vi "FipsAdjacent.vi"() -> (11 "Fips":i32[](array[numeric]))   [LabVIEW 2017] (continued)
\t33013\n\"Merrimack County, NH\"\t33013\t\"Rockingham County, NH\"\t33015\n\"Merrimack County, NH\"\t33013\t\"Strafford County, NH\"\t33017\n\"Merrimack County, NH\"\t33013\t\"Sullivan County, NH\"\t33019\n\"Rockingham County, NH\"\t33015\t\"York County, ME\"\t23031\n\"Rockingham County, NH\"\t33015\t\"Essex County, MA\"\t25009\n\"Rockingham County, NH\"\t33015\t\"Hillsborough County, NH\"\t33011\n\"Rockingham County, NH\"\t33015\t\"Merrimack County, NH\"\t33013\n\"Rockingham County, NH\"\t33015\t\"Rockingham County, NH\"\t33015\n\"Rockingham County, NH\"\t33015\t\"Strafford County, NH\"\t33017\n\"Strafford County, NH\"\t33017\t\"York County, ME\"\t23031\n\"Strafford County, NH\"\t33017\t\"Belknap County, NH\"\t33001\n\"Strafford County, NH\"\t33017\t\"Carroll County, NH\"\t33003\n\"Strafford County, NH\"\t33017\t\"Merrimack County, NH\"\t33013\n\"Strafford County, NH\"\t33017\t\"Rockingham County, NH\"\t33015\n\"Strafford County, NH\"\t33017\t\"Strafford County, NH\"\t33017\n\"Sullivan County, NH\"\t33019\t\"Cheshire County, NH\"\t33005\n\"Sullivan County, NH\"\t33019\t\"Grafton County, NH\"\t33009\n\"Sullivan County, NH\"\t33019\t\"Hillsborough County, NH\"\t33011\n\"Sullivan County, NH\"\t33019\t\"Merrimack County, NH\"\t33013\n\"Sullivan County, NH\"\t33019\t\"Sullivan County, NH\"\t33019\n\"Sullivan County, NH\"\t33019\t\"Windham County, VT\"\t50025\n\"Sullivan County, NH\"\t33019\t\"Windsor County, VT\"\t50027\n\"Atlantic County, NJ\"\t34001\t\"Atlantic County, NJ\"\t34001\n\"Atlantic County, NJ\"\t34001\t\"Burlington County, NJ\"\t34005\n\"Atlantic County, NJ\"\t34001\t\"Camden County, NJ\"\t34007\n\"Atlantic County, NJ\"\t34001\t\"Cape May County, NJ\"\t34009\n\"Atlantic County, NJ\"\t34001\t\"Cumberland County, NJ\"\t34011\n\"Atlantic County, NJ\"\t34001\t\"Gloucester County, NJ\"\t34015\n\"Atlantic County, NJ\"\t34001\t\"Ocean County, NJ\"\t34029\n\"Bergen County, NJ\"\t34003\t\"Bergen County, NJ\"\t34003\n\"Bergen County, NJ\"\t34003\t\"Essex County, NJ\"\t34013\n\"Bergen County, NJ\"\t34003\t\"Hudson County, NJ\"\t34017\n\"Bergen County, NJ\"\t34003\t\"Passaic County, NJ\"\t34031\n\"Bergen County, NJ\"\t34003\t\"Bronx County, NY\"\t36005\n\"Bergen County, NJ\"\t34003\t\"New York County, NY\"\t36061\n\"Bergen County, NJ\"\t34003\t\"Rockland County, NY\"\t36087\n\"Bergen County, NJ\"\t34003\t\"Westchester County, NY\"\t36119\n\"Burlington County, NJ\"\t34005\t\"Atlantic County, NJ\"\t34001\n\"Burlington County, NJ\"\t34005\t\"Burlington County, NJ\"\t34005\n\"Burlington County, NJ\"\t34005\t\"Camden County, NJ\"\t34007\n\"Burlington County, NJ\"\t34005\t\"Mercer County, NJ\"\t34021\n\"Burlington County, NJ\"\t34005\t\"Monmouth County, NJ\"\t34025\n\"Burlington County, NJ\"\t34005\t\"Ocean County, NJ\"\t34029\n\"Burlington County, NJ\"\t34005\t\"Bucks County, PA\"\t42017\n\"Burlington County, NJ\"\t34005\t\"Philadelphia County, PA\"\t42101\n\"Camden County, NJ\"\t34007\t\"Atlantic County, NJ\"\t34001\n\"Camden County, NJ\"\t34007\t\"Burlington County, NJ\"\t34005\n\"Camden County, NJ\"\t34007\t\"Camden County, NJ\"\t34007\n\"Camden County, NJ\"\t34007\t\"Gloucester County, NJ\"\t34015\n\"Camden County, NJ\"\t34007\t\"Philadelphia County, PA\"\t42101\n\"Cape May County, NJ\"\t34009\t\"Kent County, DE\"\t10001\n\"Cape May County, NJ\"\t34009\t\"Sussex County, DE\"\t10005\n\"Cape May County, NJ\"\t34009\t\"Atlantic County, NJ\"\t34001\n\"Cape May County, NJ\"\t34009\t\"Cape May County, NJ\"\t34009\n\"Cape May County, NJ\"\t34009\t\"Cumberland County, NJ\"\t34011\n\"Cumberland County, NJ\"\t34011\t\"Kent County, DE\"\t10001\n\"Cumberland County, NJ\"\t34011\t\"Atlantic County, NJ\"\t34001\n\"Cumberland County, NJ\"\t34011\t\"Cape May County, NJ\"\t34009\n\"Cumberland County, NJ\"\t34011\t\"Cumberland County, NJ\"\t34011\n\"Cumberland County, NJ\"\t34011\t\"Gloucester County, NJ\"\t34015\n\"Cumberland County, NJ\"\t34011\t\"Salem County, NJ\"\t34033\n\"Essex County, NJ\"\t34013\t\"Bergen County, NJ\"\t34003\n\"Essex County, NJ\"\t34013\t\"Essex County, NJ\"\t34013\n\"Essex County, NJ\"\t34013\t\"Hudson County, NJ\"\t34017\n\"Essex County, NJ\"\t34013\t\"Morris County, NJ\"\t34027\n\"Essex County, NJ\"\t34013\t\"Passaic County, NJ\"\t34031\n\"Essex County, NJ\"\t34013\t\"Union County, NJ\"\t34039\n\"Gloucester County, NJ\"\t34015\t\"New Castle County, DE\"\t10003\n\"Gloucester County, NJ\"\t34015\t\"Atlantic County, NJ\"\t34001\n\"Gloucester County, NJ\"\t34015\t\"Camden County, NJ\"\t34007\n\"Gloucester County, NJ\"\t34015\t\"Cumberland County, NJ\"\t34011\n\"Gloucester County, NJ\"\t34015\t\"Gloucester County, NJ\"\t34015\n\"Gloucester County, NJ\"\t34015\t\"Salem County, NJ\"\t34033\n\"Gloucester County, NJ\"\t34015\t\"Delaware County, PA\"\t42045\n\"Gloucester County, NJ\"\t34015\t\"Philadelphia County, PA\"\t42101\n\"Hudson County, NJ\"\t34017\t\"Bergen County, NJ\"\t34003\n\"Hudson County, NJ\"\t34017\t\"Essex County, NJ\"\t34013\n\"Hudson County, NJ\"\t34017\t\"Hudson County, NJ\"\t34017\n\"Hudson County, NJ\"\t34017\t\"Union County, NJ\"\t34039\n\"Hudson County, NJ\"\t34017\t\"Kings County, NY\"\t36047\n\"Hudson County, NJ\"\t34017\t\"New York County, NY\"\t36061\n\"Hudson County, NJ\"\t34017\t\"Richmond County, NY\"\t36085\n\"Hunterdon County, NJ\"\t34019\t\"Hunterdon County, NJ\"\t34019\n\"Hunterdon County, NJ\"\t34019\t\"Mercer County, NJ\"\t34021\n\"Hunterdon County, NJ\"\t34019\t\"Morris County, NJ\"\t34027\n\"Hunterdon County, NJ\"\t34019\t\"Somerset County, NJ\"\t34035\n\"Hunterdon County, NJ\"\t34019\t\"Warren County, NJ\"\t34041\n\"Hunterdon County, NJ\"\t34019\t\"Bucks County, PA\"\t42017\n\"Mercer County, NJ\"\t34021\t\"Burlington County, NJ\"\t34005\n\"Mercer County, NJ\"\t34021\t\"Hunterdon County, NJ\"\t34019\n\"Mercer County, NJ\"\t34021\t\"Mercer County, NJ\"\t34021\n\"Mercer County, NJ\"\t34021\t\"Middlesex County, NJ\"\t34023\n\"Mercer County, NJ\"\t34021\t\"Monmouth County, NJ\"\t34025\n\"Mercer County, NJ\"\t34021\t\"Somerset County, NJ\"\t34035\n\"Mercer County, NJ\"\t34021\t\"Bucks County, PA\"\t42017\n\"Middlesex County, NJ\"\t34023\t\"Mercer County, NJ\"\t34021\n\"Middlesex County, NJ\"\t34023\t\"Middlesex County, NJ\"\t34023\n\"Middlesex County, NJ\"\t34023\t\"Monmouth County, NJ\"\t34025\n\"Middlesex County, NJ\"\t34023\t\"Somerset County, NJ\"\t34035\n\"Middlesex County, NJ\"\t34023\t\"Union County, NJ\"\t34039\n\"Middlesex County, NJ\"\t34023\t\"Richmond County, NY\"\t36085\n\"Monmouth County, NJ\"\t34025\t\"Burlington County, NJ\"\t34005\n\"Monmouth County, NJ\"\t34025\t\"Mercer County, NJ\"\t34021\n\"Monmouth County, NJ\"\t34025\t\"Middlesex County, NJ\"\t34023\n\"Monmouth County, NJ\"\t34025\t\"Monmouth County, NJ\"\t34025\n\"Monmouth County, NJ\"\t34025\t\"Ocean County, NJ\"\t34029\n\"Monmouth County, NJ\"\t34025\t\"Queens County, NY\"\t36081\n\"Monmouth County, NJ\"\t34025\t\"Richmond County, NY\"\t36085\n\"Morris County, NJ\"\t34027\t\"Essex County, NJ\"\t34013\n\"Morris County, NJ\"\t34027\t\"Hunterdon County, NJ\"\t34019\n\"Morris County, NJ\"\t34027\t\"Morris County, NJ\"\t34027\n\"Morris County, NJ\"\t34027\t\"Passaic County, NJ\"\t34031\n\"Morris County, NJ\"\t34027\t\"Somerset County, NJ\"\t34035\n\"Morris County, NJ\"\t34027\t\"Sussex County, NJ\"\t34037\n\"Morris County, NJ\"\t34027\t\"Union County, NJ\"\t34039\n\"Morris County, NJ\"\t34027\t\"Warren County, NJ\"\t34041\n\"Ocean County, NJ\"\t34029\t\"Atlantic County, NJ\"\t34001\n\"Ocean County, NJ\"\t34029\t\"Burlington County, NJ\"\t34005\n\"Ocean County, NJ\"\t34029\t\"Monmouth County, NJ\"\t34025\n\"Ocean County, NJ\"\t34029\t\"Ocean County, NJ\"\t34029\n\"Passaic County, NJ\"\t34031\t\"Bergen County, NJ\"\t34003\n\"Passaic County, NJ\"\t34031\t\"Essex County, NJ\"\t34013\n\"Passaic County, NJ\"\t34031\t\"Morris County, NJ\"\t34027\n\"Passaic County, NJ\"\t34031\t\"Passaic County, NJ\"\t34031\n\"Passaic County, NJ\"\t34031\t\"Sussex County, NJ\"\t34037\n\"Passaic County, NJ\"\t34031\t\"Orange County, NY\"\t36071\n\"Passaic County, NJ\"\t34031\t\"Rockland County, NY\"\t36087\n\"Salem County, NJ\"\t34033\t\"Kent County, DE\"\t10001\n\"Salem County, NJ\"\t34033\t\"New Castle County, DE\"\t10003\n\"Salem County, NJ\"\t34033\t\"Cumberland County, NJ\"\t34011\n\"Salem County, NJ\"\t34033\t\"Gloucester County, NJ\"\t34015\n\"Salem County, NJ\"\t34033\t\"Salem County, NJ\"\t34033\n\"Somerset County, NJ\"\t34035\t\"Hunterdon County, NJ\"\t34019\n\"Somerset County, NJ\"\t34035\t\"Mercer County, NJ\"\t34021\n\"Somerset County, NJ\"\t34035\t\"Middlesex County, NJ\"\t34023\n\"Somerset County, NJ\"\t34035\t\"Morris County, NJ\"\t34027\n\"Somerset County, NJ\"\t34035\t\"Somerset County, NJ\"\t34035\n\"Somerset County, NJ\"\t34035\t\"Union County, NJ\"\t34039\n\"Sussex County, NJ\"\t34037\t\"Morris County, NJ\"\t34027\n\"Sussex County, NJ\"\t34037\t\"Passaic County, NJ\"\t34031\n\"Sussex County, NJ\"\t34037\t\"Sussex County, NJ\"\t34037\n\"Sussex County, NJ\"\t34037\t\"Warren County, NJ\"\t34041\n\"Sussex County, NJ\"\t34037\t\"Orange County, NY\"\t36071\n\"Sussex County, NJ\"\t34037\t\"Monroe County, PA\"\t42089\n\"Sussex County, NJ\"\t34037\t\"Pike County, PA\"\t42103\n\"Union County, NJ\"\t34039\t\"Essex County, NJ\"\t34013\n\"Union County, NJ\"\t34039\t\"Hudson County, NJ\"\t34017\n\"Union County, NJ\"\t34039\t\"Middlesex County, NJ\"\t34023\n\"Union County, NJ\"\t34039\t\"Morris County, NJ\"\t34027\n\"Union County, NJ\"\t34039\t\"Somerset County, NJ\"\t34035\n\"Union County, NJ\"\t34039\t\"Union County, NJ\"\t34039\n\"Union County, NJ\"\t34039\t\"Richmond County, NY\"\t36085\n\"Warren County, NJ\"\t34041\t\"Hunterdon County, NJ\"\t34019\n\"Warren County, NJ\"\t34041\t\"Morris County, NJ\"\t34027\n\"Warren County, NJ\"\t34041\t\"Sussex County, NJ\"\t34037\n\"Warren County, NJ\"\t34041\t\"Warren County, NJ\"\t34041\n\"Warren County, NJ\"\t34041\t\"Bucks County, PA\"\t42017\n\"Warren County, NJ\"\t34041\t\"Monroe County, PA\"\t42089\n\"Warren County, NJ\"\t34041\t\"Northampton County, PA\"\t42095\n\"Bernalillo County, NM\"\t35001\t\"Bernalillo County, NM\"\t35001\n\"Bernalillo County, NM\"\t35001\t\"Cibola County, NM\"\t35006\n\"Bernalillo County, NM\"\t35001\t\"Sandoval County, NM\"\t35043\n\"Bernalillo County, NM\"\t35001\t\"Santa Fe County, NM\"\t35049\n\"Bernalillo County, NM\"\t35001\t\"Torrance County, NM\"\t35057\n\"Bernalillo County, NM\"\t35001\t\"Valencia County, NM\"\t35061\n\"Catron County, NM\"\t35003\t\"Apache County, AZ\"\t04001\n\"Catron County, NM\"\t35003\t\"Greenlee County, AZ\"\t04011\n\"Catron County, NM\"\t35003\t\"Catron County, NM\"\t35003\n\"Catron County, NM\"\t35003\t\"Cibola County, NM\"\t35006\n\"Catron County, NM\"\t35003\t\"Grant County, NM\"\t35017\n\"Catron County, NM\"\t35003\t\"Sierra County, NM\"\t35051\n\"Catron County, NM\"\t35003\t\"Socorro County, NM\"\t35053\n\"Chaves County, NM\"\t35005\t\"Chaves County, NM\"\t35005\n\"Chaves County, NM\"\t35005\t\"De Baca County, NM\"\t35011\n\"Chaves County, NM\"\t35005\t\"Eddy County, NM\"\t35015\n\"Chaves County, NM\"\t35005\t\"Lea County, NM\"\t35025\n\"Chaves County, NM\"\t35005\t\"Lincoln County, NM\"\t35027\n\"Chaves County, NM\"\t35005\t\"Otero County, NM\"\t35035\n\"Chaves County, NM\"\t35005\t\"Roosevelt County, NM\"\t35041\n\"Cibola County, NM\"\t35006\t\"Apache County, AZ\"\t04001\n\"Cibola County, NM\"\t35006\t\"Bernalillo County, NM\"\t35001\n\"Cibola County, NM\"\t35006\t\"Catron County, NM\"\t35003\n\"Cibola County, NM\"\t35006\t\"Cibola County, NM\"\t35006\n\"Cibola County, NM\"\t35006\t\"McKinley County, NM\"\t35031\n\"Cibola County, NM\"\t35006\t\"Sandoval County, NM\"\t35043\n\"Cibola County, NM\"\t35006\t\"Socorro County, NM\"\t35053\n\"Cibola County, NM\"\t35006\t\"Valencia County, NM\"\t35061\n\"Colfax County, NM\"\t35007\t\"Costilla County, CO\"\t08023\n\"Colfax County, NM\"\t35007\t\"Las Animas County, CO\"\t08071\n\"Colfax County, NM\"\t35007\t\"Colfax County, NM\"\t35007\n\"Colfax County, NM\"\t35007\t\"Harding County, NM\"\t35021\n\"Colfax County, NM\"\t35007\t\"Mora County, NM\"\t35033\n\"Colfax County, NM\"\t35007\t\"Taos County, NM\"\t35055\n\"Colfax County, NM\"\t35007\t\"Union County, NM\"\t35059\n\"Curry County, NM\"\t35009\t\"Curry County, NM\"\t35009\n\"Curry County, NM\"\t35009\t\"Quay County, NM\"\t35037\n\"Curry County, NM\"\t35009\t\"Roosevelt County, NM\"\t35041\n\"Curry County, NM\"\t35009\t\"Bailey County, TX\"\t48017\n\"Curry County, NM\"\t35009\t\"Deaf Smith County, TX\"\t48117\n\"Curry County, NM\"\t35009\t\"Parmer County, TX\"\t48369\n\"De Baca County, NM\"\t35011\t\"Chaves County, NM\"\t35005\n\"De Baca County, NM\"\t35011\t\"De Baca County, NM\"\t35011\n\"De Baca County, NM\"\t35011\t\"Guadalupe County, NM\"\t35019\n\"De Baca County, NM\"\t35011\t\"Lincoln County, NM\"\t35027\n\"De Baca County, NM\"\t35011\t\"Quay County, NM\"\t35037\n\"De Baca County, NM\"\t35011\t\"Roosevelt County, NM\"\t35041\n\"Do?a Ana County, NM\"\t35013\t\"Do?a Ana County, NM\"\t35013\n\"Do?a Ana County, NM\"\t35013\t\"Luna County, NM\"\t35029\n\"Do?a Ana County, NM\"\t35013\t\"Otero County, NM\"\t35035\n\"Do?a Ana County, NM\"\t35013\t\"Sierra County, NM\"\t35051\n\"Do?a Ana County, NM\"\t35013\t\"El Paso County, TX\"\t48141\n\"Eddy County, NM\"\t35015\t\"Chaves County, NM\"\t35005\n\"Eddy County, NM\"\t35015\t\"Eddy County, NM\"\t35015\n\"Eddy County, NM\"\t35015\t\"Lea County, NM\"\t35025\n\"Eddy County, NM\"\t35015\t\"Otero County, NM\"\t35035\n\"Eddy County, NM\"\t35015\t\"Culberson County, TX\"\t48109\n\"Eddy County, NM\"\t35015\t\"Loving County, TX\"\t48301\n\"Eddy County, NM\"\t35015\t\"Reeves County, TX\"\t48389\n\"Grant County, NM\"\t35017\t\"Greenlee County, AZ\"\t04011\n\"Grant County, NM\"\t35017\t\"Catron County, NM\"\t35003\n\"Grant County, NM\"\t35017\t\"Grant County, NM\"\t35017\n\"Grant County, NM\"\t35017\t\"Hidalgo County, NM\"\t35023\n\"Grant County, NM\"\t35017\t\"Luna County, NM\"\t35029\n\"Grant County, NM\"\t35017\t\"Sierra County, NM\"\t35051\n\"Guadalupe County, NM\"\t35019\t\"De Baca County, NM\"\t35011\n\"Guadalupe County, NM\"\t35019\t\"Guadalupe County, NM\"\t35019\n\"Guadalupe County, NM\"\t35019\t\"Lincoln County, NM\"\t35027\n\"Guadalupe County, NM\"\t35019\t\"Quay County, NM\"\t35037\n\"Guadalupe County, NM\"\t35019\t\"San Miguel County, NM\"\t35047\n\"Guadalupe County, NM\"\t35019\t\"Torrance County, NM\"\t35057\n\"Harding County, NM\"\t35021\t\"Colfax County, NM\"\t35007\n\"Harding County, NM\"\t35021\t\"Harding County, NM\"\t35021\n\"Harding County, NM\"\t35021\t\"Mora County, NM\"\t35033\n\"Harding County, NM\"\t35021\t\"Quay County, NM\"\t35037\n\"Harding County, NM\"\t35021\t\"San Miguel County, NM\"\t35047\n\"Harding County, NM\"\t35021\t\"Union County, NM\"\t35059\n\"Hidalgo County, NM\"\t35023\t\"Cochise County, AZ\"\t04003\n\"Hidalgo County, NM\"\t35023\t\"Greenlee County, AZ\"\t04011\n\"Hidalgo County, NM\"\t35023\t\"Grant County, NM\"\t35017\n\"Hidalgo County, NM\"\t35023\t\"Hidalgo County, NM\"\t35023\n\"Hidalgo County, NM\"\t35023\t\"Luna County, NM\"\t35029\n\"Lea County, NM\"\t35025\t\"Chaves County, NM\"\t35005\n\"Lea County, NM\"\t35025\t\"Eddy County, NM\"\t35015\n\"Lea County, NM\"\t35025\t\"Lea County, NM\"\t35025\n\"Lea County, NM\"\t35025\t\"Roosevelt County, NM\"\t35041\n\"Lea County, NM\"\t35025\t\"Andrews County, TX\"\t48003\n\"Lea County, NM\"\t35025\t\"Cochran County, TX\"\t48079\n\"Lea County, NM\"\t35025\t\"Gaines County, TX\"\t48165\n\"Lea County, NM\"\t35025\t\"Loving County, TX\"\t48301\n\"Lea County, NM\"\t35025\t\"Winkler County, TX\"\t48495\n\"Lea County, NM\"\t35025\t\"Yoakum County, TX\"\t48501\n\"Lincoln County, NM\"\t35027\t\"Chaves County, NM\"\t35005\n\"Lincoln County, NM\"\t35027\t\"De Baca County, NM\"\t35011\n\"Lincoln County, NM\"\t35027\t\"Guadalupe County, NM\"\t35019\n\"Lincoln County, NM\"\t35027\t\"Lincoln County, NM\"\t35027\n\"Lincoln County, NM\"\t35027\t\"Otero County, NM\"\t35035\n\"Lincoln County, NM\"\t35027\t\"Sierra County, NM\"\t35051\n\"Lincoln County, NM\"\t35027\t\"Socorro County, NM\"\t35053\n\"Lincoln County, NM\"\t35027\t\"Torrance County, NM\"\t35057\n\"Los Alamos County, NM\"\t35028\t\"Los Alamos County, NM\"\t35028\n\"Los Alamos County, NM\"\t35028\t\"Rio Arriba County, NM\"\t35039\n\"Los Alamos County, NM\"\t35028\t\"Sandoval County, NM\"\t35043\n\"Los Alamos County, NM\"\t35028\t\"Santa Fe County, NM\"\t35049\n\"Luna County, NM\"\t35029\t\"Do?a Ana County, NM\"\t35013\n\"Luna County, NM\"\t35029\t\"Grant County, NM\"\t35017\n\"Luna County, NM\"\t35029\t\"Hidalgo County, NM\"\t35023\n\"Luna County, NM\"\t35029\t\"Luna County, NM\"\t35029\n\"Luna County, NM\"\t35029\t\"Sierra County, NM\"\t35051\n\"McKinley County, NM\"\t35031\t\"Apache County, AZ\"\t04001\n\"McKinley County, NM\"\t35031\t\"Cibola County, NM\"\t35006\n\"McKinley County, NM\"\t35031\t\"McKinley County, NM\"\t35031\n\"McKinley County, NM\"\t35031\t\"Sandoval County, NM\"\t35043\n\"McKinley County, NM\"\t35031\t\"San Juan County, NM\"\t35045\n\"Mora County, NM\"\t35033\t\"Colfax County, NM\"\t35007\n\"Mora County, NM\"\t35033\t\"Harding County, NM\"\t35021\n\"Mora County, NM\"\t35033\t\"Mora County, NM\"\t35033\n\"Mora County, NM\"\t35033\t\"Rio Arriba County, NM\"\t35039\n\"Mora County, NM\"\t35033\t\"San Miguel County, NM\"\t35047\n\"Mora County, NM\"\t35033\t\"Santa Fe County, NM\"\t35049\n\"Mora County, NM\"\t35033\t\"Taos County, NM\"\t35055\n\"Otero County, NM\"\t35035\t\"Chaves County, NM\"\t35005\n\"Otero County, NM\"\t35035\t\"Do?a Ana County, NM\"\t35013\n\"Otero County, NM\"\t35035\t\"Eddy County, NM\"\t35015\n\"Otero County, NM\"\t35035\t\"Lincoln County, NM\"\t35027\n\"Otero County, NM\"\t35035\t\"Otero County, NM\"\t35035\n\"Otero County, NM\"\t35035\t\"Sierra County, NM\"\t35051\n\"Otero County, NM\"\t35035\t\"Culberson County, TX\"\t48109\n\"Otero County, NM\"\t35035\t\"El Paso County, TX\"\t48141\n\"Otero County, NM\"\t35035\t\"Hudspeth County, TX\"\t48229\n\"Quay County, NM\"\t35037\t\"Curry County, NM\"\t35009\n\"Quay County, NM\"\t35037\t\"De Baca County, NM\"\t35011\n\"Quay County, NM\"\t35037\t\"Guadalupe County, NM\"\t35019\n\"Quay County, NM\"\t35037\t\"Harding County, NM\"\t35021\n\"Quay County, NM\"\t35037\t\"Quay County, NM\"\t35037\n\"Quay County, NM\"\t35037\t\"Roosevelt County, NM\"\t35041\n\"Quay County, NM\"\t35037\t\"San Miguel County, NM\"\t35047\n\"Quay County, NM\"\t35037\t\"Union County, NM\"\t35059\n\"Quay County, NM\"\t35037\t\"Deaf Smith County, TX\"\t48117\n\"Quay County, NM\"\t35037\t\"Hartley County, TX\"\t48205\n\"Quay County, NM\"\t35037\t\"Oldham County, TX\"\t48359\n\"Rio Arriba County, NM\"\t35039\t\"Archuleta County, CO\"\t08007\n\"Rio Arriba County, NM\"\t35039\t\"Conejos County, CO\"\t08021\n\"Rio Arriba County, NM\"\t35039\t\"Los Alamos County, NM\"\t35028\n\"Rio Arriba County, NM\"\t35039\t\"Mora County, NM\"\t35033\n\"Rio Arriba County, NM\"\t35039\t\"Rio Arriba County, NM\"\t35039\n\"Rio Arriba County, NM\"\t35039\t\"Sandoval County, NM\"\t35043\n\"Rio Arriba County, NM\"\t35039\t\"San Juan County, NM\"\t35045\n\"Rio Arriba County, NM\"\t35039\t\"Santa Fe County, NM\"\t35049\n\"Rio Arriba County, NM\"\t35039\t\"Taos County, NM\"\t35055\n\"Roosevelt County, NM\"\t35041\t\"Chaves County, NM\"\t35005\n\"Roosevelt County, NM\"\t35041\t\"Curry County, NM\"\t35009\n\"Roosevelt County, NM\"\t35041\t\"De Baca County, NM\"\t35011\n\"Roosevelt County, NM\"\t35041\t\"Lea County, NM\"\t35025\n\"Roosevelt County, NM\"\t35041\t\"Quay County, NM\"\t35037\n\"Roosevelt County, NM\"\t35041\t\"Roosevelt County, NM\"\t35041\n\"Roosevelt County, NM\"\t35041\t\"Bailey County, TX\"\t48017\n\"Roosevelt County, NM\"\t35041\t\"Cochran County, TX\"\t48079\n\"Sandoval County, NM\"\t35043\t\"Bernalillo County, NM\"\t35001\n\"Sandoval County, NM\"\t35043\t\"Cibola County, NM\"\t35006\n\"Sandoval County, NM\"\t35043\t\"Los Alamos County, NM\"\t35028\n\"Sandoval County, NM\"\t35043\t\"McKinley County, NM\"\t35031\n\"Sandoval County, NM\"\t35043\t\"Rio Arriba County, NM\"\t35039\n\"Sandoval County, NM\"\t35043\t\"Sandoval County, NM\"\t35043\n\"Sandoval County, NM\"\t35043\t\"San Juan County, NM\"\t35045\n\"Sandoval County, NM\"\t35043\t\"Santa Fe County, NM\"\t35049\n\"San Juan County, NM\"\t35045\t\"Apache County, AZ\"\t04001\n\"San Juan County, NM\"\t35045\t\"Archuleta County, CO\"\t08007\n\"San Juan County, NM\"\t35045\t\"La Plata County, CO\"\t08067\n\"San Juan County, NM\"\t35045\t\"Montezuma County, CO\"\t08083\n\"San Juan County, NM\"\t35045\t\"McKinley County, NM\"\t35031\n\"San Juan County, NM\"\t35045\t\"Rio Arriba County, NM\"\t35039\n\"San Juan County, NM\"\t35045\t\"Sandoval County, NM\"\t35043\n\"San Juan County, NM\"\t35045\t\"San Juan County, NM\"\t35045\n\"San Juan County, NM\"\t35045\t\"San Juan County, UT\"\t49037\n\"San Miguel County, NM\"\t35047\t\"Guadalupe County, NM\"\t35019\n\"San Miguel County, NM\"\t35047\t\"Harding County, NM\"\t35021\n\"San Miguel County, NM\"\t35047\t\"Mora County, NM\"\t35033\n\"San Miguel County, NM\"\t35047\t\"Quay County, NM\"\t35037\n\"San Miguel County, NM\"\t35047\t\"San Miguel County, NM\"\t35047\n\"San Miguel County, NM\"\t35047\t\"Santa Fe County, NM\"\t35049\n\"San Miguel County, NM\"\t35047\t\"Torrance County, NM\"\t35057\n\"Santa Fe County, NM\"\t35049\t\"Bernalillo County, NM\"\t35001\n\"Santa Fe County, NM\"\t35049\t\"Los Alamos County, NM\"\t35028\n\"Santa Fe County, NM\"\t35049\t\"Mora County, NM\"\t35033\n\"Santa Fe County, NM\"\t35049\t\"Rio Arriba County, NM\"\t35039\n\"Santa Fe County, NM\"\t35049\t\"Sandoval County, NM\"\t35043\n\"Santa Fe County, NM\"\t35049\t\"San Miguel County, NM\"\t35047\n\"Santa Fe County, NM\"\t35049\t\"Santa Fe County, NM\"\t35049\n\"Santa Fe County, NM\"\t35049\t\"Torrance County, NM\"\t35057\n\"Sierra County, NM\"\t35051\t\"Catron County, NM\"\t35003\n\"Sierra County, NM\"\t35051\t\"Do?a Ana County, NM\"\t35013\n\"Sierra County, NM\"\t35051\t\"Grant County, NM\"\t35017\n\"Sierra County, NM\"\t35051\t\"Lincoln County, NM\"\t35027\n\"Sierra County, NM\"\t35051\t\"Luna County, NM\"\t35029\n\"Sierra County, NM\"\t35051\t\"Otero County, NM\"\t35035\n\"Sierra County, NM\"\t35051\t\"Sierra County, NM\"\t35051\n\"Sierra County, NM\"\t35051\t\"Socorro County, NM\"\t35053\n\"Socorro County, NM\"\t35053\t\"Catron County, NM\"\t35003\n\"Socorro County, NM\"\t35053\t\"Cibola County, NM\"\t35006\n\"Socorro County, NM\"\t35053\t\"Lincoln County, NM\"\t35027\n\"Socorro County, NM\"\t35053\t\"Sierra County, NM\"\t35051\n\"Socorro County, NM\"\t35053\t\"Socorro County, NM\"\t35053\n\"Socorro County, NM\"\t35053\t\"Torrance County, NM\"\t35057\n\"Socorro County, NM\"\t35053\t\"Valencia County, NM\"\t35061\n\"Taos County, NM\"\t35055\t\"Conejos County, CO\"\t08021\n\"Taos County, NM\"\t35055\t\"Costilla County, CO\"\t08023\n\"Taos County, NM\"\t35055\t\"Colfax County, NM\"\t35007\n\"Taos County, NM\"\t35055\t\"Mora County, NM\"\t35033\n\"Taos County, NM\"\t35055\t\"Rio Arriba County, NM\"\t35039\n\"Taos County, NM\"\t35055\t\"Taos County, NM\"\t35055\n\"Torrance County, NM\"\t35057\t\"Bernalillo County, NM\"\t35001\n\"Torrance County, NM\"\t35057\t\"Guadalupe County, NM\"\t35019\n\"Torrance County, NM\"\t35057\t\"Lincoln County, NM\"\t35027\n\"Torrance County, NM\"\t35057\t\"San Miguel County, NM\"\t35047\n\"Torrance County, NM\"\t35057\t\"Santa Fe County, NM\"\t35049\n\"Torrance County, NM\"\t35057\t\"Socorro County, NM\"\t35053\n\"Torrance County, NM\"\t35057\t\"Torrance County, NM\"\t35057\n\"Torrance County, NM\"\t35057\t\"Valencia County, NM\"\t35061\n\"Union County, NM\"\t35059\t\"Baca County, CO\"\t08009\n\"Union County, NM\"\t35059\t\"Las Animas County, CO\"\t08071\n\"Union County, NM\"\t35059\t\"Colfax County, NM\"\t35007\n\"Union County, NM\"\t35059\t\"Harding County, NM\"\t35021\n\"Union County, NM\"\t35059\t\"Quay County, NM\"\t35037\n\"Union County, NM\"\t35059\t\"Union County, NM\"\t35059\n\"Union County, NM\"\t35059\t\"Cimarron County, OK\"\t40025\n\"Union County, NM\"\t35059\t\"Dallam County, TX\"\t48111\n\"Union County, NM\"\t35059\t\"Hartley County, TX\"\t48205\n\"Valencia County, NM\"\t35061\t\"Bernalillo County, NM\"\t35001\n\"Valencia County, NM\"\t35061\t\"Cibola County, NM\"\t35006\n\"Valencia County, NM\"\t35061\t\"Socorro County, NM\"\t35053\n\"Valencia County, NM\"\t35061\t\"Torrance County, NM\"\t35057\n\"Valencia County, NM\"\t35061\t\"Valencia County, NM\"\t35061\n\"Albany County, NY\"\t36001\t\"Albany County, NY\"\t36001\n\"Albany County, NY\"\t36001\t\"Columbia County, NY\"\t36021\n\"Albany County, NY\"\t36001\t\"Greene County, NY\"\t36039\n\"Albany County, NY\"\t36001\t\"Rensselaer County, NY\"\t36083\n\"Albany County, NY\"\t36001\t\"Saratoga County, NY\"\t36091\n\"Albany County, NY\"\t36001\t\"Schenectady County, NY\"\t36093\n\"Albany County, NY\"\t36001\t\"Schoharie County, NY\"\t36095\n\"Allegany County, NY\"\t36003\t\"Allegany County, NY\"\t36003\n\"Allegany County, NY\"\t36003\t\"Cattaraugus County, NY\"\t36009\n\"Allegany County, NY\"\t36003\t\"Livingston County, NY\"\t36051\n\"Allegany County, NY\"\t36003\t\"Steuben County, NY\"\t36101\n\"Allegany County, NY\"\t36003\t\"Wyoming County, NY\"\t36121\n\"Allegany County, NY\"\t36003\t\"McKean County, PA\"\t42083\n\"Allegany County, NY\"\t36003\t\"Potter County, PA\"\t42105\n\"Bronx County, NY\"\t36005\t\"Bergen County, NJ\"\t34003\n\"Bronx County, NY\"\t36005\t\"Bronx County, NY\"\t36005\n\"Bronx County, NY\"\t36005\t\"Nassau County, NY\"\t36059\n\"Bronx County, NY\"\t36005\t\"New York County, NY\"\t36061\n\"Bronx County, NY\"\t36005\t\"Queens County, NY\"\t36081\n\"Bronx County, NY\"\t36005\t\"Westchester County, NY\"\t36119\n\"Broome County, NY\"\t36007\t\"Broome County, NY\"\t36007\n\"Broome County, NY\"\t36007\t\"Chenango County, NY\"\t36017\n\"Broome County, NY\"\t36007\t\"Cortland County, NY\"\t36023\n\"Broome County, NY\"\t36007\t\"Delaware County, NY\"\t36025\n\"Broome County, NY\"\t36007\t\"Tioga County, NY\"\t36107\n\"Broome County, NY\"\t36007\t\"Susquehanna County, PA\"\t42115\n\"Broome County, NY\"\t36007\t\"Wayne County, PA\"\t42127\n\"Cattaraugus County, NY\"\t36009\t\"Allegany County, NY\"\t36003\n\"Cattaraugus County, NY\"\t36009\t\"Cattaraugus County, NY\"\t36009\n\"Cattaraugus County, NY\"\t36009\t\"Chautauqua County, NY\"\t36013\n\"Cattaraugus County, NY\"\t36009\t\"Erie County, NY\"\t36029\n\"Cattaraugus County, NY\"\t36009\t\"Wyoming County, NY\"\t36121\n\"Cattaraugus County, NY\"\t36009\t\"McKean County, PA\"\t42083\n\"Cattaraugus County, NY\"\t36009\t\"Warren County, PA\"\t42123\n\"Cayuga County, NY\"\t36011\t\"Cayuga County, NY\"\t36011\n\"Cayuga County, NY\"\t36011\t\"Cortland County, NY\"\t36023\n\"Cayuga County, NY\"\t36011\t\"Jefferson County, NY\"\t36045\n\"Cayuga County, NY\"\t36011\t\"Onondaga County, NY\"\t36067\n\"Cayuga County, NY\"\t36011\t\"Oswego County, NY\"\t36075\n\"Cayuga County, NY\"\t36011\t\"Seneca County, NY\"\t36099\n\"Cayuga County, NY\"\t36011\t\"Tompkins County, NY\"\t36109\n\"Cayuga County, NY\"\t36011\t\"Wayne County, NY\"\t36117\n\"Chautauqua County, NY\"\t36013\t\"Cattaraugus County, NY\"\t36009\n\"Chautauqua County, NY\"\t36013\t\"Chautauqua County, NY\"\t36013\n\"Chautauqua County, NY\"\t36013\t\"Erie County, NY\"\t36029\n\"Chautauqua County, NY\"\t36013\t\"Erie County, PA\"\t42049\n\"Chautauqua County, NY\"\t36013\t\"Warren County, PA\"\t42123\n\"Chemung County, NY\"\t36015\t\"Chemung County, NY\"\t36015\n\"Chemung County, NY\"\t36015\t\"Schuyler County, NY\"\t36097\n\"Chemung County, NY\"\t36015\t\"Steuben County, NY\"\t36101\n\"Chemung County, NY\"\t36015\t\"Tioga County, NY\"\t36107\n\"Chemung County, NY\"\t36015\t\"Tompkins County, NY\"\t36109\n\"Chemung County, NY\"\t36015\t\"Bradford County, PA\"\t42015\n\"Chemung County, NY\"\t36015\t\"Tioga County, PA\"\t42117\n\"Chenango County, NY\"\t36017\t\"Broome County, NY\"\t36007\n\"Chenango County, NY\"\t36017\t\"Chenango County, NY\"\t36017\n\"Chenango County, NY\"\t36017\t\"Cortland County, NY\"\t36023\n\"Chenango County, NY\"\t36017\t\"Delaware County, NY\"\t36025\n\"Chenango County, NY\"\t36017\t\"Madison County, NY\"\t36053\n\"Chenango County, NY\"\t36017\t\"Otsego County, NY\"\t36077\n\"Clinton County, NY\"\t36019\t\"Clinton County, NY\"\t36019\n\"Clinton County, NY\"\t36019\t\"Essex County, NY\"\t36031\n\"Clinton County, NY\"\t36019\t\"Franklin County, NY\"\t36033\n\"Clinton County, NY\"\t36019\t\"Chittenden County, VT\"\t50007\n\"Clinton County, NY\"\t36019\t\"Grand Isle County, VT\"\t50013\n\"Columbia County, NY\"\t36021\t\"Berkshire County, MA\"\t25003\n\"Columbia County, NY\"\t36021\t\"Albany County, NY\"\t36001\n\"Columbia County, NY\"\t36021\t\"Columbia County, NY\"\t36021\n\"Columbia County, NY\"\t36021\t\"Dutchess County, NY\"\t36027\n\"Columbia County, NY\"\t36021\t\"Greene County, NY\"\t36039\n\"Columbia County, NY\"\t36021\t\"Rensselaer County, NY\"\t36083\n\"Columbia County, NY\"\t36021\t\"Ulster County, NY\"\t36111\n\"Cortland County, NY\"\t36023\t\"Broome County, NY\"\t36007\n\"Cortland County, NY\"\t36023\t\"Cayuga County, NY\"\t36011\n\"Cortland County, NY\"\t36023\t\"Chenango County, NY\"\t36017\n\"Cortland County, NY\"\t36023\t\"Cortland County, NY\"\t36023\n\"Cortland County, NY\"\t36023\t\"Madison County, NY\"\t36053\n\"Cortland County, NY\"\t36023\t\"Onondaga County, NY\"\t36067\n\"Cortland County, NY\"\t36023\t\"Tioga County, NY\"\t36107\n\"Cortland County, NY\"\t36023\t\"Tompkins County, NY\"\t36109\n\"Delaware County, NY\"\t36025\t\"Broome County, NY\"\t36007\n\"Delaware County, NY\"\t36025\t\"Chenango County, NY\"\t36017\n\"Delaware County, NY\"\t36025\t\"Delaware County, NY\"\t36025\n\"Delaware County, NY\"\t36025\t\"Greene County, NY\"\t36039\n\"Delaware County, NY\"\t36025\t\"Otsego County, NY\"\t36077\n\"Delaware County, NY\"\t36025\t\"Schoharie County, NY\"\t36095\n\"Delaware County, NY\"\t36025\t\"Sullivan County, NY\"\t36105\n\"Delaware County, NY\"\t36025\t\"Ulster County, NY\"\t36111\n\"Delaware County, NY\"\t36025\t\"Wayne County, PA\"\t42127\n\"Dutchess County, NY\"\t36027\t\"Fairfield County, CT\"\t09001\n\"Dutchess County, NY\"\t36027\t\"Litchfield County, CT\"\t09005\n\"Dutchess County, NY\"\t36027\t\"Berkshire County, MA\"\t25003\n\"Dutchess County, NY\"\t36027\t\"Columbia County, NY\"\t36021\n\"Dutchess County, NY\"\t36027\t\"Dutchess County, NY\"\t36027\n\"Dutchess County, NY\"\t36027\t\"Orange County, NY\"\t36071\n\"Dutchess County, NY\"\t36027\t\"Putnam County, NY\"\t36079\n\"Dutchess County, NY\"\t36027\t\"Ulster County, NY\"\t36111\n\"Erie County, NY\"\t36029\t\"Cattaraugus County, NY\"\t36009\n\"Erie County, NY\"\t36029\t\"Chautauqua County, NY\"\t36013\n\"Erie County, NY\"\t36029\t\"Erie County, NY\"\t36029\n\"Erie County, NY\"\t36029\t\"Genesee County, NY\"\t36037\n\"Erie County, NY\"\t36029\t\"Niagara County, NY\"\t36063\n\"Erie County, NY\"\t36029\t\"Wyoming County, NY\"\t36121\n\"Essex County, NY\"\t36031\t\"Clinton County, NY\"\t36019\n\"Essex County, NY\"\t36031\t\"Essex County, NY\"\t36031\n\"Essex County, NY\"\t36031\t\"Franklin County, NY\"\t36033\n\"Essex County, NY\"\t36031\t\"Hamilton County, NY\"\t36041\n\"Essex County, NY\"\t36031\t\"Warren County, NY\"\t36113\n\"Essex County, NY\"\t36031\t\"Washington County, NY\"\t36115\n\"Essex County, NY\"\t36031\t\"Addison County, VT\"\t50001\n\"Essex County, NY\"\t36031\t\"Chittenden County, VT\"\t50007\n\"Franklin County, NY\"\t36033\t\"Clinton County, NY\"\t36019\n\"Franklin County, NY\"\t36033\t\"Essex County, NY\"\t36031\n\"Franklin County, NY\"\t36033\t\"Franklin County, NY\"\t36033\n\"Franklin County, NY\"\t36033\t\"Hamilton County, NY\"\t36041\n\"Franklin County, NY\"\t36033\t\"St. Lawrence County, NY\"\t36089\n\"Fulton County, NY\"\t36035\t\"Fulton County, NY\"\t36035\n\"Fulton County, NY\"\t36035\t\"Hamilton County, NY\"\t36041\n\"Fulton County, NY\"\t36035\t\"Herkimer County, NY\"\t36043\n\"Fulton County, NY\"\t36035\t\"Montgomery County, NY\"\t36057\n\"Fulton County, NY\"\t36035\t\"Saratoga County, NY\"\t36091\n\"Genesee County, NY\"\t36037\t\"Erie County, NY\"\t36029\n\"Genesee County, NY\"\t36037\t\"Genesee County, NY\"\t36037\n\"Genesee County, NY\"\t36037\t\"Livingston County, NY\"\t36051\n\"Genesee County, NY\"\t36037\t\"Monroe County, NY\"\t36055\n\"Genesee County, NY\"\t36037\t\"Niagara County, NY\"\t36063\n\"Genesee County, NY\"\t36037\t\"Orleans County, NY\"\t36073\n\"Genesee County, NY\"\t36037\t\"Wyoming County, NY\"\t36121\n\"Greene County, NY\"\t36039\t\"Albany County, NY\"\t36001\n\"Greene County, NY\"\t36039\t\"Columbia County, NY\"\t36021\n\"Greene County, NY\"\t36039\t\"Delaware County, NY\"\t36025\n\"Greene County, NY\"\t36039\t\"Greene County, NY\"\t36039\n\"Greene County, NY\"\t36039\t\"Rensselaer County, NY\"\t36083\n\"Greene County, NY\"\t36039\t\"Schoharie County, NY\"\t36095\n\"Greene County, NY\"\t36039\t\"Ulster County, NY\"\t36111\n\"Hamilton County, NY\"\t36041\t\"Essex County, NY\"\t36031\n\"Hamilton County, NY\"\t36041\t\"Franklin County, NY\"\t36033\n\"Hamilton County, NY\"\t36041\t\"Fulton County, NY\"\t36035\n\"Hamilton County, NY\"\t36041\t\"Hamilton County, NY\"\t36041\n\"Hamilton County, NY\"\t36041\t\"Herkimer County, NY\"\t36043\n\"Hamilton County, NY\"\t36041\t\"St. Lawrence County, NY\"\t36089\n\"Hamilton County, NY\"\t36041\t\"Saratoga County, NY\"\t36091\n\"Hamilton County, NY\"\t36041\t\"Warren County, NY\"\t36113\n\"Herkimer County, NY\"\t36043\t\"Fulton County, NY\"\t36035\n\"Herkimer County, NY\"\t36043\t\"Hamilton County, NY\"\t36041\n\"Herkimer County, NY\"\t36043\t\"Herkimer County, NY\"\t36043\n\"Herkimer County, NY\"\t36043\t\"Lewis County, NY\"\t36049\n\"Herkimer County, NY\"\t36043\t\"Montgomery County, NY\"\t36057\n\"Herkimer County, NY\"\t36043\t\"Oneida County, NY\"\t36065\n\"Herkimer County, NY\"\t36043\t\"Otsego County, NY\"\t36077\n\"Herkimer County, NY\"\t36043\t\"St. Lawrence County, NY\"\t36089\n\"Jefferson County, NY\"\t36045\t\"Cayuga County, NY\"\t36011\n\"Jefferson County, NY\"\t36045\t\"Jefferson County, NY\"\t36045\n\"Jefferson County, NY\"\t36045\t\"Lewis County, NY\"\t36049\n\"Jefferson County, NY\"\t36045\t\"Oswego County, NY\"\t36075\n\"Jefferson County, NY\"\t36045\t\"St. Lawrence County, NY\"\t36089\n\"Kings County, NY\"\t36047\t\"Hudson County, NJ\"\t34017\n\"Kings County, NY\"\t36047\t\"Kings County, NY\"\t36047\n\"Kings County, NY\"\t36047\t\"New York County, NY\"\t36061\n\"Kings County, NY\"\t36047\t\"Queens County, NY\"\t36081\n\"Kings County, NY\"\t36047\t\"Richmond County, NY\"\t36085\n\"Lewis County, NY\"\t36049\t\"Herkimer County, NY\"\t36043\n\"Lewis County, NY\"\t36049\t\"Jefferson County, NY\"\t36045\n\"Lewis County, NY\"\t36049\t\"Lewis County, NY\"\t36049\n\"Lewis County, NY\"\t36049\t\"Oneida County, NY\"\t36065\n\"Lewis County, NY\"\t36049\t\"Oswego County, NY\"\t36075\n\"Lewis County, NY\"\t36049\t\"St. Lawrence County, NY\"\t36089\n\"Livingston County, NY\"\t36051\t\"Allegany County, NY\"\t36003\n\"Livingston County, NY\"\t36051\t\"Genesee County, NY\"\t36037\n\"Livingston County, NY\"\t36051\t\"Livingston County, NY\"\t36051\n\"Livingston County, NY\"\t36051\t\"Monroe County, NY\"\t36055\n\"Livingston County, NY\"\t36051\t\"Ontario County, NY\"\t36069\n\"Livingston County, NY\"\t36051\t\"Steuben County, NY\"\t36101\n\"Livingston County, NY\"\t36051\t\"Wyoming County, NY\"\t36121\n\"Madison County, NY\"\t36053\t\"Chenango County, NY\"\t36017\n\"Madison County, NY\"\t36053\t\"Cortland County, NY\"\t36023\n\"Madison County, NY\"\t36053\t\"Madison County, NY\"\t36053\n\"Madison County, NY\"\t36053\t\"Oneida County, NY\"\t36065\n\"Madison County, NY\"\t36053\t\"Onondaga County, NY\"\t36067\n\"Madison County, NY\"\t36053\t\"Oswego County, NY\"\t36075\n\"Madison County, NY\"\t36053\t\"Otsego County, NY\"\t36077\n\"Monroe County, NY\"\t36055\t\"Genesee County, NY\"\t36037\n\"Monroe County, NY\"\t36055\t\"Livingston County, NY\"\t36051\n\"Monroe County, NY\"\t36055\t\"Monroe County, NY\"\t36055\n\"Monroe County, NY\"\t36055\t\"Ontario County, NY\"\t36069\n\"Monroe County, NY\"\t36055\t\"Orleans County, NY\"\t36073\n\"Monroe County, NY\"\t36055\t\"Wayne County, NY\"\t36117\n\"Montgomery County, NY\"\t36057\t\"Fulton County, NY\"\t36035\n\"Montgomery County, NY\"\t36057\t\"Herkimer County, NY\"\t36043\n\"Montgomery County, NY\"\t36057\t\"Montgomery County, NY\"\t36057\n\"Montgomery County, NY\"\t36057\t\"Otsego County, NY\"\t36077\n\"Montgomery County, NY\"\t36057\t\"Saratoga County, NY\"\t36091\n\"Montgomery County, NY\"\t36057\t\"Schenectady County, NY\"\t36093\n\"Montgomery County, NY\"\t36057\t\"Schoharie County, NY\"\t36095\n\"Nassau County, NY\"\t36059\t\"Fairfield County, CT\"\t09001\n\"Nassau County, NY\"\t36059\t\"Bronx County, NY\"\t36005\n\"Nassau County, NY\"\t36059\t\"Nassau County, NY\"\t36059\n\"Nassau County, NY\"\t36059\t\"Queens County, NY\"\t36081\n\"Nassau County, NY\"\t36059\t\"Suffolk County, NY\"\t36103\n\"Nassau County, NY\"\t36059\t\"Westchester County, NY\"\t36119\n\"New York County, NY\"\t36061\t\"Bergen County, NJ\"\t34003\n\"New York County, NY\"\t36061\t\"Hudson County, NJ\"\t34017\n\"New York County, NY\"\t36061\t\"Bronx County, NY\"\t36005\n\"New York County, NY\"\t36061\t\"Kings County, NY\"\t36047\n\"New York County, NY\"\t36061\t\"New York County, NY\"\t36061\n\"New York County, NY\"\t36061\t\"Queens County, NY\"\t36081\n\"Niagara County, NY\"\t36063\t\"Erie County, NY\"\t36029\n\"Niagara County, NY\"\t36063\t\"Genesee County, NY\"\t36037\n\"Niagara County, NY\"\t36063\t\"Niagara County, NY\"\t36063\n\"Niagara County, NY\"\t36063\t\"Orleans County, NY\"\t36073\n\"Oneida County, NY\"\t36065\t\"Herkimer County, NY\"\t36043\n\"Oneida County, NY\"\t36065\t\"Lewis County, NY\"\t36049\n\"Oneida County, NY\"\t36065\t\"Madison County, NY\"\t36053\n\"Oneida County, NY\"\t36065\t\"Oneida County, NY\"\t36065\n\"Oneida County, NY\"\t36065\t\"Oswego County, NY\"\t36075\n\"Oneida County, NY\"\t36065\t\"Otsego County, NY\"\t36077\n\"Onondaga County, NY\"\t36067\t\"Cayuga County, NY\"\t36011\n\"Onondaga County, NY\"\t36067\t\"Cortland County, NY\"\t36023\n\"Onondaga County, NY\"\t36067\t\"Madison County, NY\"\t36053\n\"Onondaga County, NY\"\t36067\t\"Onondaga County, NY\"\t36067\n\"Onondaga County, NY\"\t36067\t\"Oswego County, NY\"\t36075\n\"Ontario County, NY\"\t36069\t\"Livingston County, NY\"\t36051\n\"Ontario County, NY\"\t36069\t\"Monroe County, NY\"\t36055\n\"Ontario County, NY\"\t36069\t\"Ontario County, NY\"\t36069\n\"Ontario County, NY\"\t36069\t\"Seneca County, NY\"\t36099\n\"Ontario County, NY\"\t36069\t\"Steuben County, NY\"\t36101\n\"Ontario County, NY\"\t36069\t\"Wayne County, NY\"\t36117\n\"Ontario County, NY\"\t36069\t\"Yates County, NY\"\t36123\n\"Orange County, NY\"\t36071\t\"Passaic County, NJ\"\t34031\n\"Orange County, NY\"\t36071\t\"Sussex County, NJ\"\t34037\n\"Orange County, NY\"\t36071\t\"Dutchess County, NY\"\t36027\n\"Orange County, NY\"\t36071\t\"Orange County, NY\"\t36071\n\"Orange County, NY\"\t36071\t\"Putnam County, NY\"\t36079\n\"Orange County, NY\"\t36071\t\"Rockland County, NY\"\t36087\n\"Orange County, NY\"\t36071\t\"Sullivan County, NY\"\t36105\n\"Orange County, NY\"\t36071\t\"Ulster County, NY\"\t36111\n\"Orange County, NY\"\t36071\t\"Pike County, PA\"\t42103\n\"Orleans County, NY\"\t36073\t\"Genesee County, NY\"\t36037\n\"Orleans County, NY\"\t36073\t\"Monroe County, NY\"\t36055\n\"Orleans County, NY\"\t36073\t\"Niagara County, NY\"\t36063\n\"Orleans County, NY\"\t36073\t\"Orleans County, NY\"\t36073\n\"Oswego County, NY\"\t36075\t\"Cayuga County, NY\"\t36011\n\"Oswego County, NY\"\t36075\t\"Jefferson County, NY\"\t36045\n\"Oswego County, NY\"\t36075\t\"Lewis County, NY\"\t36049\n\"Oswego County, NY\"\t36075\t\"Madison County, NY\"\t36053\n\"Oswego County, NY\"\t36075\t\"Oneida County, NY\"\t36065\n\"Oswego County, NY\"\t36075\t\"Onondaga County, NY\"\t36067\n\"Oswego County, NY\"\t36075\t\"Oswego County, NY\"\t36075\n\"Otsego County, NY\"\t36077\t\"Chenango County, NY\"\t36017\n\"Otsego County, NY\"\t36077\t\"Delaware County, NY\"\t36025\n\"Otsego County, NY\"\t36077\t\"Herkimer County, NY\"\t36043\n\"Otsego County, NY
